vi "RenumberGraphCrv.vi"(8 "error in (no error)":errorcluster caption="entrée d'erreur (pas d'erreur)", 10 "AllCurves":string[](array[string]), 11 "Interface en entrée":refnum<class "Interface.lvclass"> caption="DNL_LabVIEW Object in") -> (0 "error out":errorcluster caption="sortie d'erreur", 3 "Interface en sortie":refnum<class "Interface.lvclass"> caption="DNL_LabVIEW Object out")   [LabVIEW 2019, in "Interface.lvclass"]
uses:
  Interface.lvclass
  Interface.lvclass/Interface.ctl
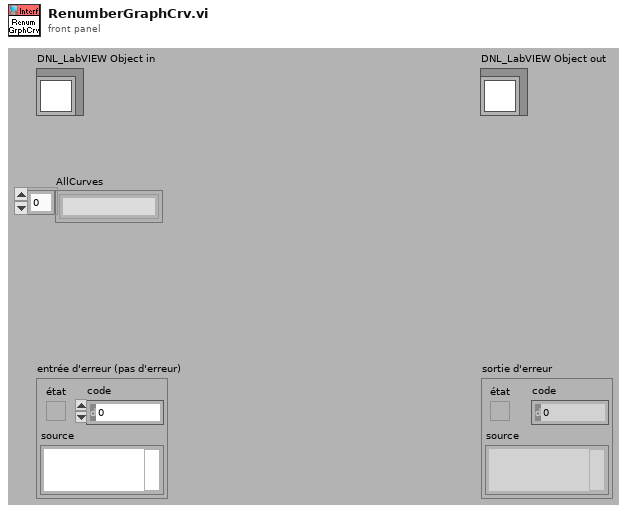
[diagram p1: front panel]
types:
  T1 = typedef "Interface.lvclass/CurveSetup.ctl" = cluster{"CurveName":string, "YParam":string, "XParam":string, "ZParam ":string, "GroupName":string, "LinWdth":u8, "PntCol":u32, "LinCol":u32, "LablFor":u8, "XScale":u32, "YScale":u32, "Interpol":u8, "DisplayName":string, "FillType":i16, "LineStyle":u8, "PntStyle":u8, "BarTyp":u8, "GraphIndex":i32, "Visible":bool, "XScaleName":string, "YScaleName":string, "XYGraph_Ref":refnum<vi>, "Data Only":bool, "DataQ Ref":refnum<queue>, "XParQ Ref":refnum<queue>, "XParamInd":i32, "ScanInd":i32, "File Path":path}
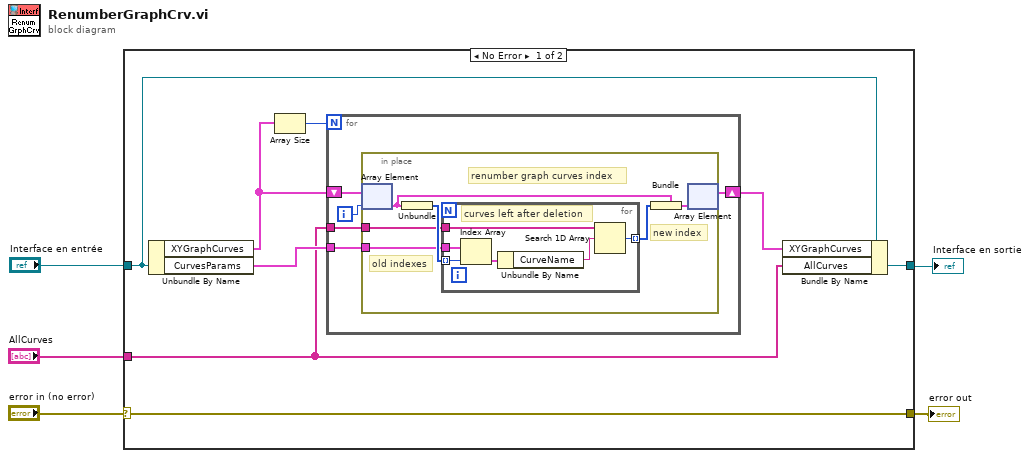
[diagram p0: block diagram]
diagram:
  n1 = case shown="No Error" "error in (no error)" {
    selector: "error in (no error)" -> [w8 w32]
    tunnel: [w8 w32] -> w4
    tunnel: [w13 w31] -> w2
    tunnel: "Interface en entrée" -> [w12 w31]
    tunnel: "AllCurves" -> [w7 _]
    frame No Error {
      n2 = Unbundle By Name(w12) -> ("XYGraphCurves"=w6:cluster{"Tableau":i32[]}[], "CurvesParams"=w9:T1[])
      n3 = Array Size(array=w6) -> (size(s)=w11:i32)
      n4 = for {
        N: w11 -> [_]
        shift-right: [w14] -> w10
        shift-left: w6 -> [w18]
        tunnel: w9 -> [w16]
        tunnel: w7 -> [w15]
        i -> [w17]
        n5 = in-place {
          in-place-border: w16 -> [w23]
          in-place-border: w15 -> [w22]
          # "old indexes"
          # "new index"
          # "renumber graph curves index"
          n6 = in-place-array #1(w18, w17) -> (w21:cluster{"Tableau":i32[]})
          n7 = Unbundle(w21) -> ("Tableau"=w24:i32[])
          n8 = for {
            tunnel: w24 -> [w30] mode=indexing
            tunnel: w23 -> [w29]
            tunnel: w22 -> [w26]
            tunnel: [w25] -> w19 mode=indexing
            # "curves left after deletion"
            n9 = Index Array(array=w29, index=w30) -> (element=w28:T1)
            n10 = Unbundle By Name(w28) -> ("CurveName"=w27:string)
            n11 = Search 1D Array(1D array=w26, element=w27) -> (index of element=w25:i32)  [unwired: 1 in]
          }
          n12 = Bundle(cluster=w21, "Tableau"=w19) -> (w20:cluster{"Tableau":i32[]})
          n13 = in-place-array #1(w20) -> (w14:cluster{"Tableau":i32[]}[])  [unwired: 1 out]
        }
      }
      n14 = Bundle By Name(cluster=w12, "XYGraphCurves"=w10, "AllCurves"=w7) -> (w13:refnum<class "Interface.lvclass">)
    }
    frame Error {
    }
  }
  "error out" <- w4
  "Interface en sortie" <- w2
